vi "VITester_Global_OnCommand.vi"(10 "Command ID":string, 11 "Object":T1) -> ()   [LabVIEW 2009]
uses:
  Support/VITester Project Item Ref.ctl
  <vilib>/addons/_JKI Toolkits/VI Tester/VI Tester API.llb/VI Tester API.lvlib
  <vilib>/addons/_JKI Toolkits/VI Tester/VI Tester API.llb/Run Tests (Path).vi
  <vilib>/addons/_JKI Toolkits/VI Tester/VI Tester Project API.llb/VI Tester Project API.lvlib
  Support/VI Tester Project API Method Selector - Enum.ctl
panel:
  out "error out":errorcluster
  in  "error in":errorcluster
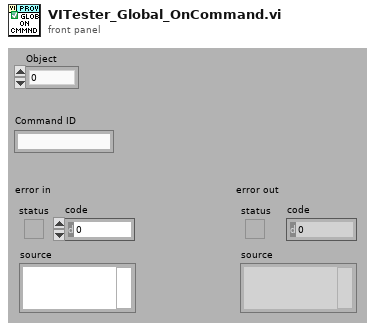
[diagram p1: front panel]
types:
  T1 = typedef "VITester Project Item Ref.ctl" = u64
  T2 = typedef "VI Tester Project API Method Selector - Enum.ctl" = enum16{"Open VI Tester", "Run All Tests", "Create New TestCase", "Create New TestSuite"}
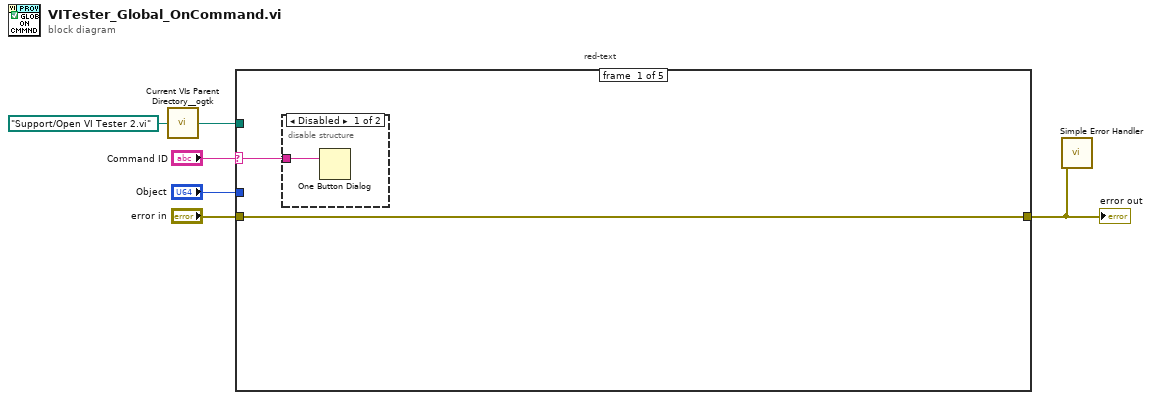
[diagram p0: block diagram]
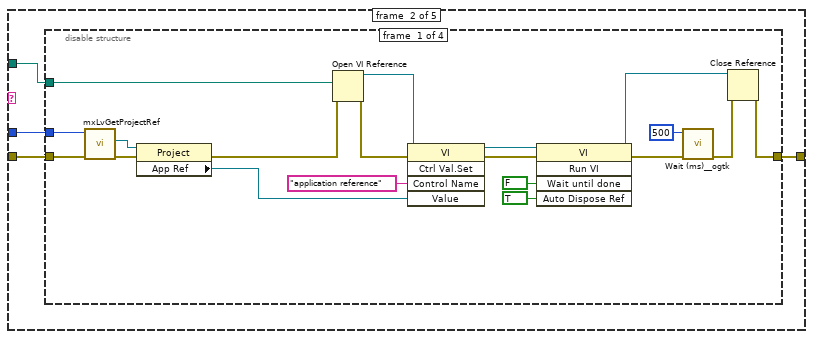
[diagram p3: hidden frame]
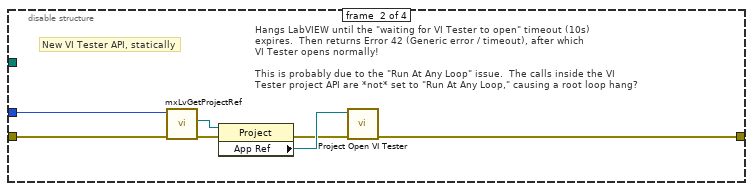
[diagram p4: hidden frame]
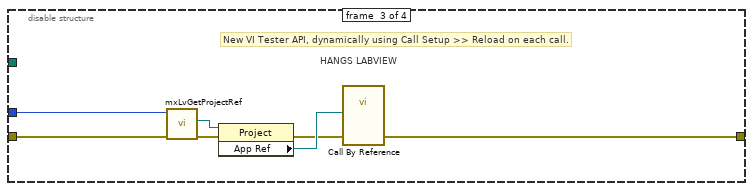
[diagram p5: hidden frame]
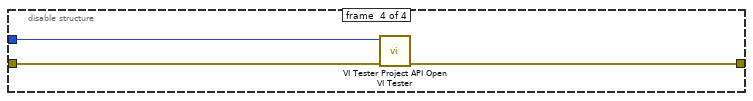
[diagram p6: hidden frame]
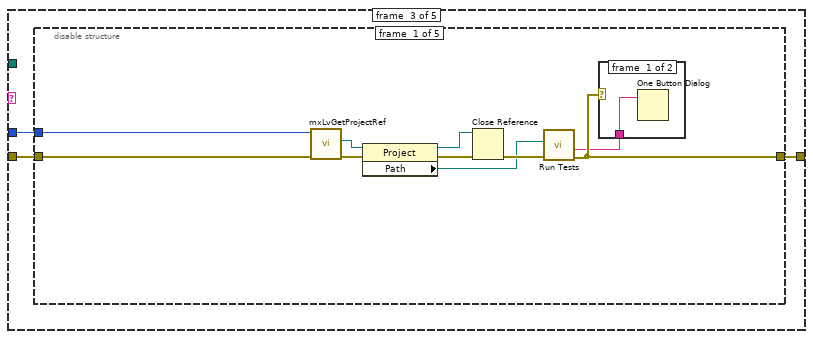
[diagram p7: hidden frame]
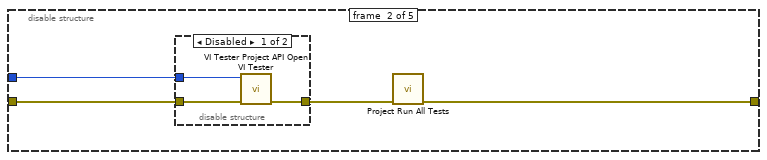
[diagram p9: hidden frame]
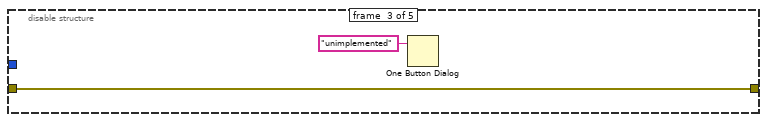
[diagram p11: hidden frame]
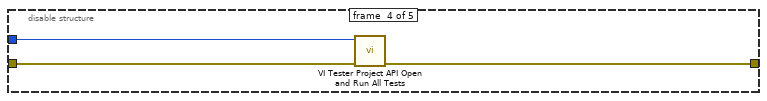
[diagram p12: hidden frame]
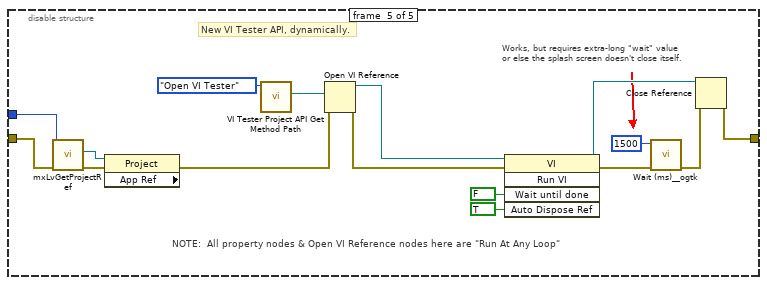
[diagram p13: hidden frame]
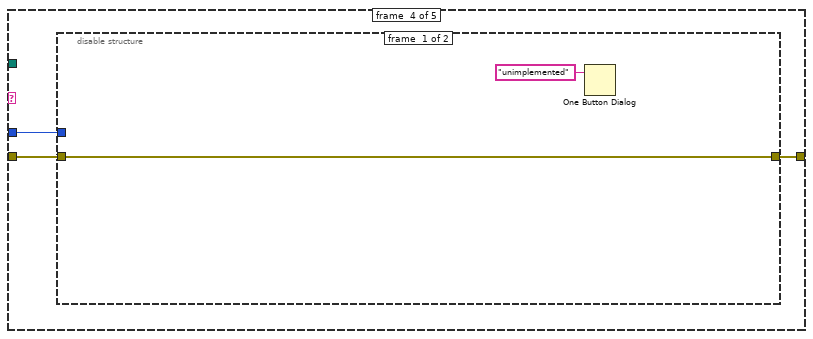
[diagram p14: hidden frame]
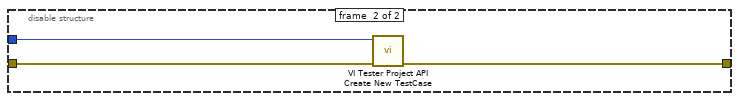
[diagram p15: hidden frame]
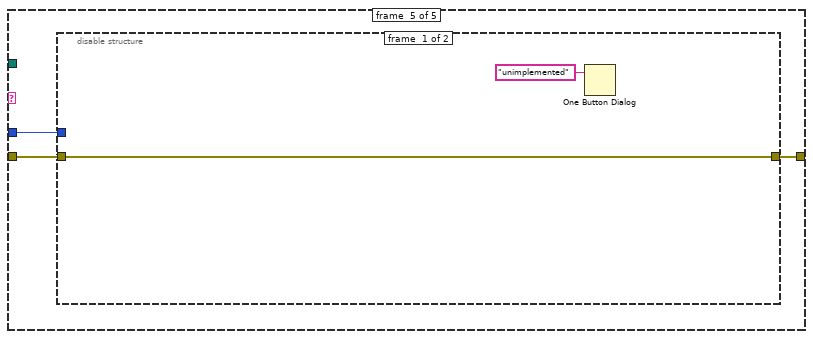
[diagram p16: hidden frame]
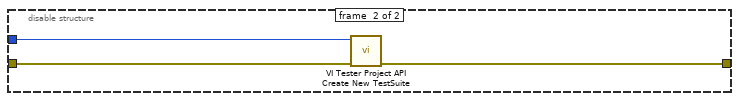
[diagram p17: hidden frame]
diagram:
  # "red-text"
  n1 = call <userlib>:"Current VIs Parent Directory__ogtk.vi"("Relative path (.)"=path "Support/Open VI Tester 2.vi") -> ("Parent Directory (+ Relative)"=w3:path)  [unwired: 4 in]
  n2 = case shown="\"TOOLBAR_RUN_ALL_TESTS\"" "Command ID" {
    selector: "Command ID" -> [w8 _ _ _ _]
    tunnel: "error in" -> [w7 w12 w52 w94 w102]
    tunnel: [w7 w11 w50 w95 w103] -> w1
    tunnel: "Object" -> [_ w10 w51 w93 w101]
    tunnel: w3 -> [_ w13 _ _ _]
    frame #0 {
      n3 = disable-structure shown="Disabled" {
        disable-tunnel: w8 -> [w9 _]
        frame #0 {
          n4 = One Button Dialog(message=w9) -> ()  [unwired: 1 in, 1 out]
        }
        frame #1 {
        }
      }
    }
    frame #1 {
      n5 = disable-structure shown="Enabled" {
        disable-tunnel: w13 -> [w32 _ _ _]
        disable-tunnel: w12 -> [w16 w36 w43 w49]
        disable-tunnel: [w28 w35 w42 w47] -> w11
        disable-tunnel: w10 -> [w18 w33 w40 w48]
        frame #0 {
          n6 = call "mxLvGetProjectRef.vi"("error in"=w16, "Item"=w18) -> ("error out"=w17:errorcluster, "Project Refnum"=w19:refnum<vi>)  [unwired: 7 in, 1 out]
          n7 = property class="Project"(reference=w19, error in=w17) -> (error out=w15:errorcluster, "App Ref"=w14:refnum<vi>)  [unwired: 1 out]
          n8 = Open VI Reference(vi path=w32, error in (no error)=w15) -> (vi reference=w22:refnum<vi>, error out=w24:errorcluster)  [unwired: 4 in]
          n9 = invoke class="VI" method="Ctrl Val.Set"(reference=w22, error in=w24, "Control Name"="application reference", "Value"=w14) -> (reference out=w21:refnum<vi>, error out=w23:errorcluster)  [unwired: 1 in, 3 out]
          n10 = invoke class="VI" method="Run VI"(reference=w21, error in=w23, "Wait until done"=FALSE ("Wait Until Done"), "Auto Dispose Ref"=TRUE ("Auto Dispose Reference")) -> (reference out=w31:refnum<vi>, error out=w27:errorcluster)  [unwired: 1 in, 3 out]
          n11 = call <userlib>:"Wait (ms)__ogtk.vi"("error in (no error)"=w27, "milliseconds to wait"=u32 500) -> ("error out"=w26:errorcluster)  [unwired: 8 in, 1 out]
          n12 = Close Reference(reference=w31, error in (no error)=w26) -> (error out=w28:errorcluster)
        }
        frame #1 {
          # "Hangs LabVIEW until the \"waiting for VI Tester to open\" timeout (10s)\nexpires.  Then returns Error 42 (Generic error / timeout), after which\nVI Tester opens normally!\n\nThis is probably due to the \"Run At Any Loop\" issue.  The calls inside the VI\nTester project API are *not* set to \"Run At Any Loop,\" causing a root loop hang?"
          # "New VI Tester API, statically"
          n13 = call "mxLvGetProjectRef.vi"("error in"=w36, "Item"=w33) -> ("error out"=w39:errorcluster, "Project Refnum"=w38:refnum<vi>)  [unwired: 7 in, 1 out]
          n14 = property class="Project"(reference=w38, error in=w39) -> (error out=w34:errorcluster, "App Ref"=w37:refnum<vi>)  [unwired: 1 out]
          n15 = call <vilib>:"Project Open VI Tester.vi"("error in (no error)"=w34, "application reference (This Application)"=w37) -> ("error out"=w35:errorcluster)  [unwired: 9 in]
        }
        frame #2 {
          # "HANGS LABVIEW"
          # "New VI Tester API, dynamically using Call Setup >> Reload on each call."
          n16 = call "mxLvGetProjectRef.vi"("error in"=w43, "Item"=w40) -> ("error out"=w46:errorcluster, "Project Refnum"=w45:refnum<vi>)  [unwired: 7 in, 1 out]
          n17 = property class="Project"(reference=w45, error in=w46) -> (error out=w41:errorcluster, "App Ref"=w44:refnum<vi>)  [unwired: 1 out]
          n18 = call-by-ref "?"("error in (no error)"=w41, "application reference"=w44) -> ("error out"=w42:errorcluster)  [unwired: 11 in, 2 out]
        }
        frame #3 {
          n19 = call "VI Tester Project API Open VI Tester.vi"("error in"=w49, "Object"=w48) -> ("error out"=w47:errorcluster)  [unwired: 9 in]
        }
      }
    }
    frame #2 {
      n20 = disable-structure shown="Enabled" {
        disable-tunnel: w52 -> [w61 w66 w72 w76 w83]
        disable-tunnel: w51 -> [w58 w67 _ w74 w82]
        disable-tunnel: [w54 w64 w72 w75 w81] -> w50
        frame #0 {
          n21 = call "mxLvGetProjectRef.vi"("error in"=w61, "Item"=w58) -> ("error out"=w60:errorcluster, "Project Refnum"=w57:refnum<vi>)  [unwired: 7 in, 1 out]
          n22 = property class="Project"(reference=w57, error in=w60) -> (reference out=w62:refnum<vi>, error out=w59:errorcluster, "Path"=w55:path)
          n23 = Close Reference(reference=w62, error in (no error)=w59) -> (error out=w56:errorcluster)
          n24 = call-poly <vilib>:"Run Tests.vi"("error in (no error)"=w56, "Test Path"=w55) -> ("error out"=w54:errorcluster, "test details"=w53:string)  [unwired: 7 in, 1 out]
          n25 = case shown="No Error" w54 {
            tunnel: w53 -> [w63 _]
            frame #0 {
              n26 = One Button Dialog(message=w63) -> ()  [unwired: 1 in, 1 out]
            }
            frame #1 {
            }
          }
        }
        frame #1 {
          n27 = disable-structure shown="Disabled" {
            disable-tunnel: w67 -> [w70 _]
            disable-tunnel: w66 -> [w69 w71]
            disable-tunnel: [w68 w71] -> w65
            frame #0 {
              n28 = call "VI Tester Project API Open VI Tester.vi"("error in"=w69, "Object"=w70) -> ("error out"=w68:errorcluster)  [unwired: 9 in]
            }
            frame #1 {
            }
          }
          n29 = call <vilib>:"Project Run All Tests.vi"("error in (no error)"=w65) -> ("error out"=w64:errorcluster)  [unwired: 10 in]
        }
        frame #2 {
          n30 = One Button Dialog(message="unimplemented") -> ()  [unwired: 1 in, 1 out]
        }
        frame #3 {
          n31 = call "VI Tester Project API Open and Run All Tests.vi"("error in"=w76, "Object"=w74) -> ("error out"=w75:errorcluster)  [unwired: 9 in]
        }
        frame #4 {
          # "Works, but requires extra-long \"wait\" value\nor else the splash screen doesn't close itself."
          # "NOTE:  All property nodes & Open VI Reference nodes here are \"Run At Any Loop\""
          # "New VI Tester API, dynamically."
          n32 = call "mxLvGetProjectRef.vi"("error in"=w83, "Item"=w82) -> ("error out"=w85:errorcluster, "Project Refnum"=w86:refnum<vi>)  [unwired: 7 in, 1 out]
          n33 = property class="Project" props=["App Ref"](reference=w86, error in=w85) -> (error out=w84:errorcluster)  [unwired: 2 out]
          n34 = call "VI Tester Project API Get Method Path.vi"("Project API Method"=VI_Tester_Project_API_Method_Selector_-_Enum."Open VI Tester") -> ("Path to VI Tester Project API Proxy VI"=w79:path)  [unwired: 9 in, 1 out]
          n35 = Open VI Reference(vi path=w79, error in (no error)=w84) -> (vi reference=w77:refnum<vi>, error out=w78:errorcluster)  [unwired: 4 in]
          n36 = invoke class="VI" method="Run VI"(reference=w77, error in=w78, "Wait until done"=FALSE ("Wait Until Done"), "Auto Dispose Ref"=TRUE ("Auto Dispose Reference")) -> (reference out=w92:refnum<vi>, error out=w88:errorcluster)  [unwired: 1 in, 3 out]
          n37 = call <userlib>:"Wait (ms)__ogtk.vi"("error in (no error)"=w88, "milliseconds to wait"=u32 1500) -> ("error out"=w91:errorcluster)  [unwired: 8 in, 1 out]
          n38 = Close Reference(reference=w92, error in (no error)=w91) -> (error out=w81:errorcluster)
        }
      }
    }
    frame #3 {
      n39 = disable-structure shown="Enabled" {
        disable-tunnel: [w96 w99] -> w95
        disable-tunnel: w94 -> [w96 w100]
        disable-tunnel: w93 -> [_ w98]
        frame #0 {
          n40 = One Button Dialog(message="unimplemented") -> ()  [unwired: 1 in, 1 out]
        }
        frame #1 {
          n41 = call "VI Tester Project API Create New TestCase.vi"("error in"=w100, "Object"=w98) -> ("error out"=w99:errorcluster)  [unwired: 9 in]
        }
      }
    }
    frame #4 {
      n42 = disable-structure shown="Enabled" {
        disable-tunnel: [w104 w106] -> w103
        disable-tunnel: w102 -> [w104 w107]
        disable-tunnel: w101 -> [_ w108]
        frame #0 {
          n43 = One Button Dialog(message="unimplemented") -> ()  [unwired: 1 in, 1 out]
        }
        frame #1 {
          n44 = call "VI Tester Project API Create New TestSuite.vi"("error in"=w107, "Object"=w108) -> ("error out"=w106:errorcluster)  [unwired: 9 in]
        }
      }
    }
  }
  "error out" <- w1
  n45 = call <vilib>:"Simple Error Handler.vi"("error in (no error)"=w1) -> ()  [unwired: 4 in, 5 out]
